vi "Sort2DArrayByCol.vi"(9 "Sort Column":i32, 10 "Current Selected Row":i32, 11 "ItemNames":string[][](array[string])) -> (2 "Sorted Selected Row":i32, 3 "Reversed 2D Array":string[][](array[string]))   [LabVIEW 2013]
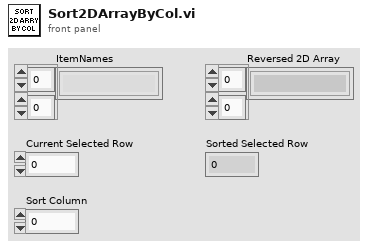
[diagram p1: front panel]
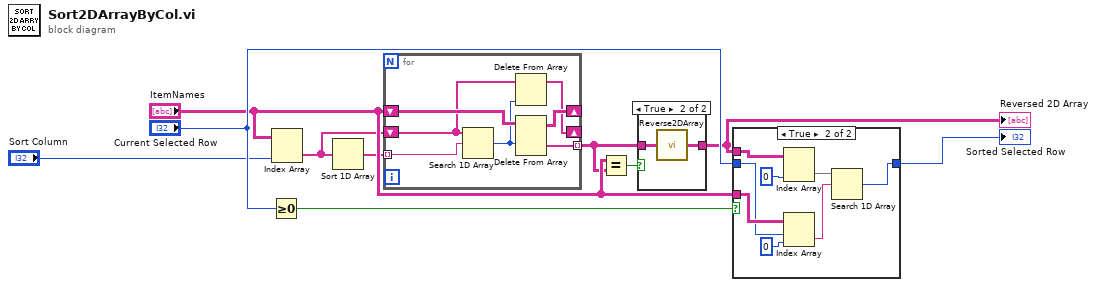
[diagram p0: block diagram]
diagram:
  n1 = Greater Or Equal To 0?(x="Current Selected Row") -> (x >= 0?=w8:bool)
  n2 = Index Array(array="ItemNames", index (col)="Sort Column") -> (element=w3:string[])  [unwired: 1 in]
  n3 = Sort 1D Array(array=w3) -> (sorted array=w2:string[])
  n4 = for {
    shift-right: [w16] -> _
    shift-left: "ItemNames" -> [w17]
    tunnel: w2 -> [w13] mode=indexing
    shift-right: [w15] -> _
    shift-left: w3 -> [w14]
    tunnel: [w11] -> w5 mode=indexing
    n5 = Search 1D Array(1D array=w14, element=w13) -> (index of element=w12:i32)  [unwired: 1 in]
    n6 = Delete From Array(array=w14, index=w12) -> (array with subset deleted=w15:string[])  [unwired: 1 in, 1 out]
    n7 = Delete From Array(array=w17, index (row)=w12) -> (deleted portion=w11:string[], array with subset deleted=w16:string[][])  [unwired: 2 in]
  }
  n8 = Equal?(x="ItemNames", y=w5) -> (x = y?=w4:bool)
  n9 = case shown="True" w4 {
    tunnel: w5 -> [w18 w20]
    tunnel: [w18 w19] -> w7
    frame False {
    }
    frame True {
      n10 = call "Reverse2DArray.vi"("2D Array"=w20) -> ("Reversed 2D Array"=w19:string[][])
    }
  }
  "Reversed 2D Array" <- w7
  n11 = case shown="True" w8 {
    tunnel: "ItemNames" -> [_ w29]
    tunnel: w7 -> [_ w26]
    tunnel: "Current Selected Row" -> [w21 w28]
    tunnel: [w21 w22] -> w9
    frame False {
    }
    frame True {
      n12 = Index Array(array=w26, index (col)=0 ("disabled index (col)")) -> (element=w24:string[])  [unwired: 1 in]
      n13 = Index Array(array=w29, index (row)=w28, index (col)=0 ("disabled index (col)")) -> (element=w23:string)
      n14 = Search 1D Array(1D array=w24, element=w23) -> (index of element=w22:i32)  [unwired: 1 in]
    }
  }
  "Sorted Selected Row" <- w9
